vi "BioFeedback12(DoubleEnvelope)-BROKEN.vi"(7 "Frames Per Second":dbl=30.0, 9 "Start Trial":bool, 11 "End Trial":bool, 12 "Data Directory":path, 13 "File Name":string, 14 "Extension":string="_EMG.txt") -> ()   [LabVIEW 2016]
uses:
  <vilib>/Utility/error.llb/DialogType.ctl
  <vilib>/Waveform/WDTOps.llb/WDT Append Waveforms DBL.vi
  <vilib>/Waveform/WDTFileIO.llb/Export Waveforms To Spreadsheet File (1D).vi
  <vilib>/Utility/file.llb/Write Delimited Spreadsheet (string).vi
panel:
  out "frames":dbl
  out "RmsBuffers 2":dbl[][](array[numeric])
  out "rmsBuffersForChannel":dbl[](array[numeric])
  out "romsToAdd":dbl
  out "PrevRMS":dbl
  out "FilteredTrialData":waveform(dbl)[](graph)
  out "FilteredAndRectified":waveform(dbl)[](graph) caption="Filtered and Rectified"
  out "FilteredTrialData":waveform(dbl)[](array[waveform])
  in  "DisplayChannel":dbl
  out "DisplayTrialData":dbl[][](array[numeric])
  out "RMSAverageByChannel":dbl[](array[numeric])
  out "DispBufferSize":dbl
  out "DispBufferIndices":dbl[](array[numeric])
  in  "Big Window Length (s)":dbl=0.5
  out "DisplayBuffers":dbl[][](array[numeric])
  out "ProcessedTrialData":dbl[][](array[numeric])
  out "CurrentRMSByChannel":dbl[](array[numeric])
  out "RmsBuffers":dbl[][](array[numeric])
  out "Trial Data Column Headers":string[](array[string])
  in  "TrialDataRowHeaders":string[](array[string])=["Wfm1", "Wfm2", "Wfm3", "Wfm4", "Wfm5", "Wfm6", "Wfm7", "Wfm8"]
  out "GetMaxStartTime":timestamp
  in  "SecondsToAcquireMax":dbl=10.0
  in  "NumberOfMaximumsToTake":dbl=3.0
  in  "CurrentMaxIndex":dbl
  out "SignalsMaxArray":dbl[](array[numeric])
  out "SignalMaxTrialsArray":dbl[][](array[numeric])
  in  "%StdDevIndex":dbl=5.0
  in  "Mean%Index":dbl=4.0
  in  "StdDevIndex":dbl=3.0
  in  "MeanIndex":dbl=2.0
  in  "MaxIndex":dbl=1.0
  in  "MinIndex":dbl
  out "Stability Data":dbl[][](array[numeric])
  out "RawTrialData":waveform(dbl)[](array[waveform])
  in  "UI Ampl Error Path":path=path "C:/Users/Tinggroup/Desktop/VRMuscleActivationVisualizer/VRBiofeedback_v2/assets/BiofeedbackAmplitudeError.txt"
  out "DisplayActivation":dbl
  out "Acquiring Max":bool
  in  "resetMax":bool
  in  "startGetMax":bool
  in  "Amplitude Error":dbl
  in  "UI Data Path":path=path "C:/Users/Tinggroup/Desktop/VRMuscleActivationVisualizer/VRBiofeedback_v2/assets/LeftEMGData.txt"
  in  "EMG Input Device\nProduct Type":string="USB-6009"
  out "DisplayBarActivation":dbl(slide) caption="Left" max=1.0 scale=0.0..100.0
  out "Processed8":dbl[](graph)
  out "Processsed7":dbl[](graph)
  out "Processed6":dbl[](graph)
  out "Processed5":dbl[](graph)
  out "Processed4":dbl[](graph)
  out "Processed3":dbl[](graph)
  out "Processed2":dbl[](graph)
  out "Processed1":dbl[](graph)
  out "Raw Trial Data Wfm":waveform(dbl)[](graph)
  in  "UI Percent Path":path=path "C:/Users/Tinggroup/Desktop/VRMuscleActivationVisualizer/VRBiofeedback_v2/assets/BiofeedbackTargetPercentage.txt"
  in  "Target Percentage":dbl=10.0
  out "Trial In Progress":bool
  in  "Lower Cut-Off":dbl=20.0
  in  "Upper Cut-Off":dbl=300.0
  out "raw data":dynamicdata(graph)
  out "RmsBufferIndices":dbl[](array[numeric])
  out "RMSBufferSize":dbl
  out "Samples per frame":dbl
  out "Reset Data Acquisition\nAnd UI Updating":bool=TRUE
  in  "Small Window Length (s)":dbl=0.5
  in  "Sample rate (Hz)":dbl=2000.0
  in  "End Program":bool
  # "Saving Trial Data"
  # "Filter and Process Parameters"
  # "Set Target"
  # "Changes are made instantly and cause moving average to reset to zero"
  # "Scale Max"
  # "Channels used in Display"
  # "Analyze Stability of Displayed Data"
  # "Auto Analyze Stability begins calculating stability\nAs soon as dot enters the target zone and stops \nonce the dot leaves the target zone (Not Yet Implemented)"
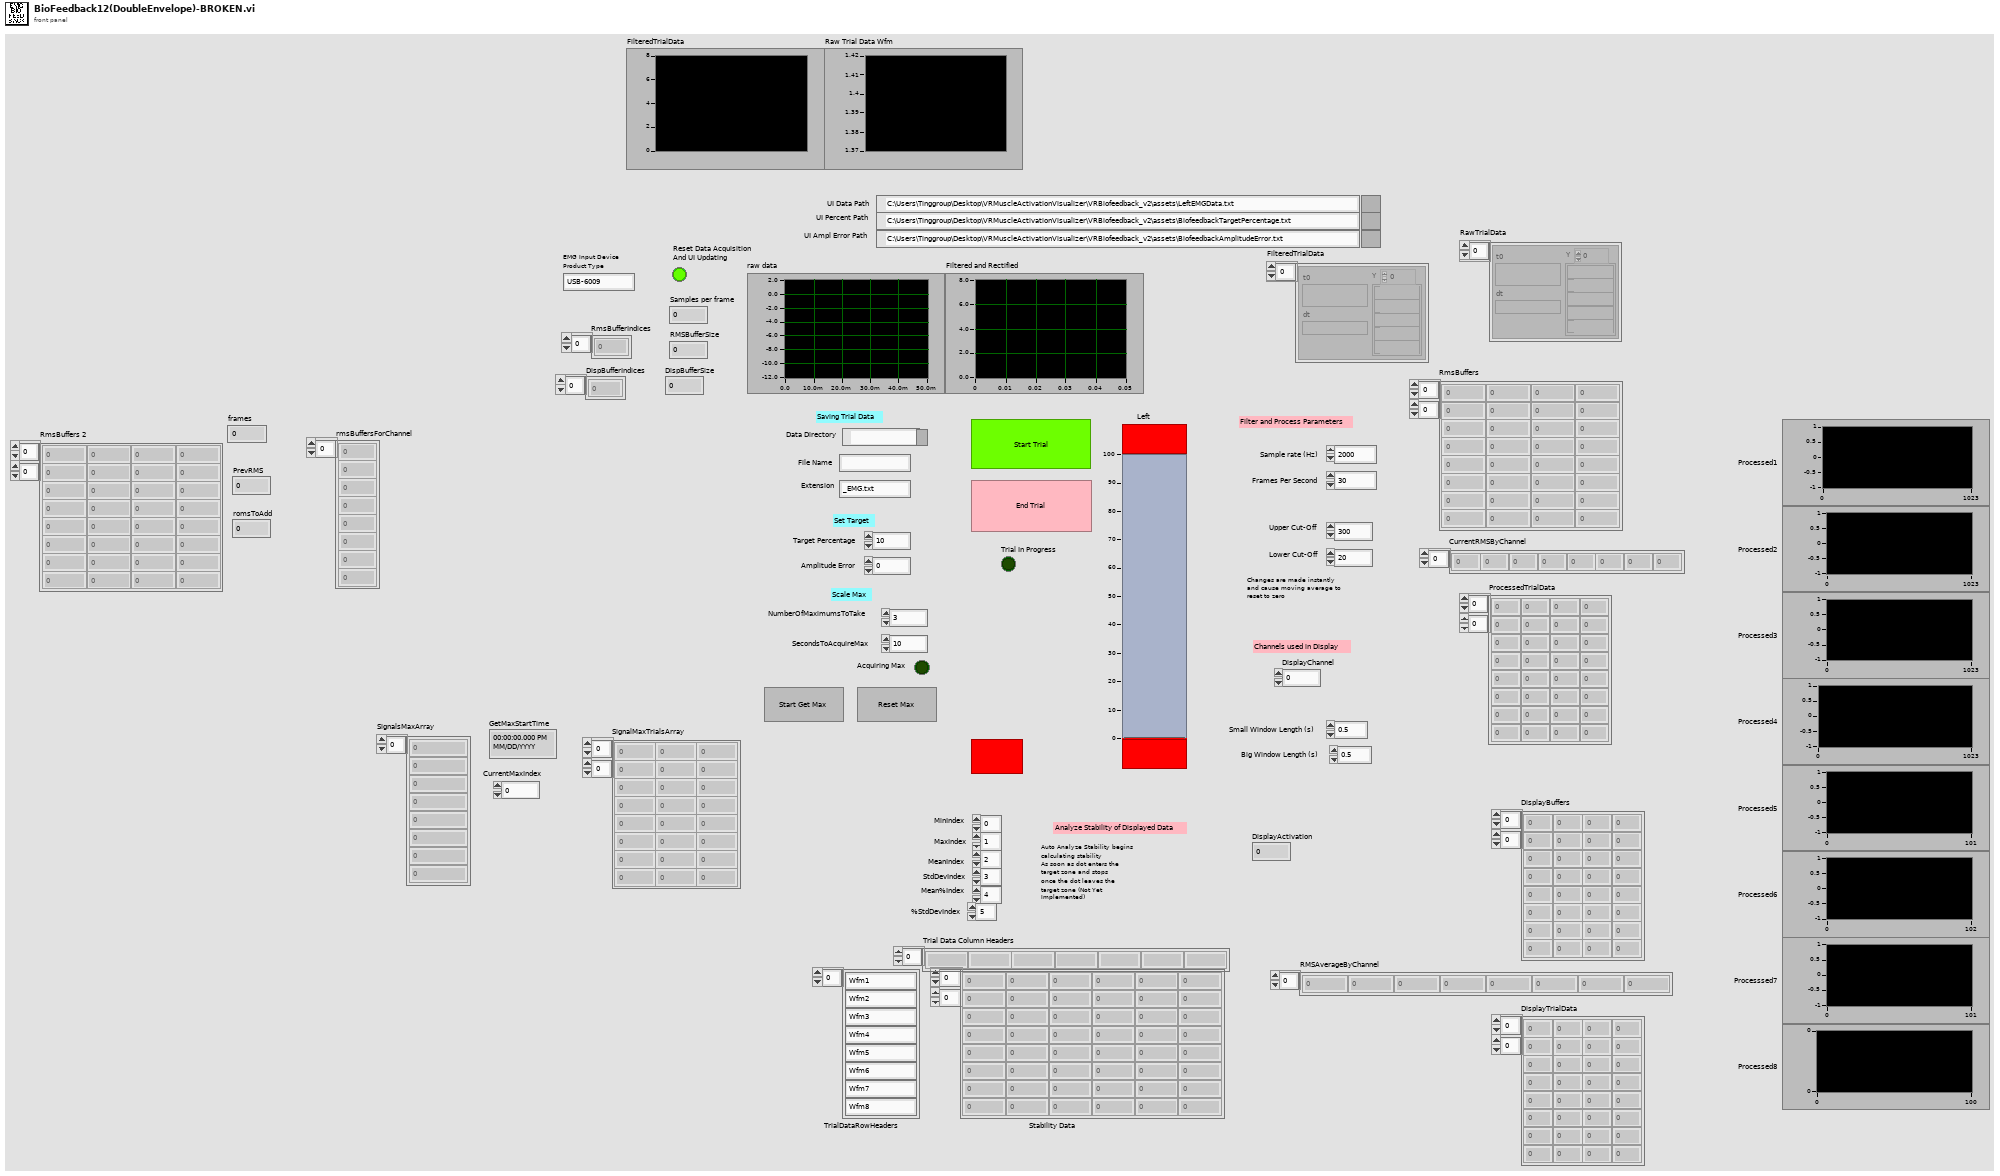
[diagram p1: front panel]
types:
  T1 = typedef "DialogType.ctl" = u16
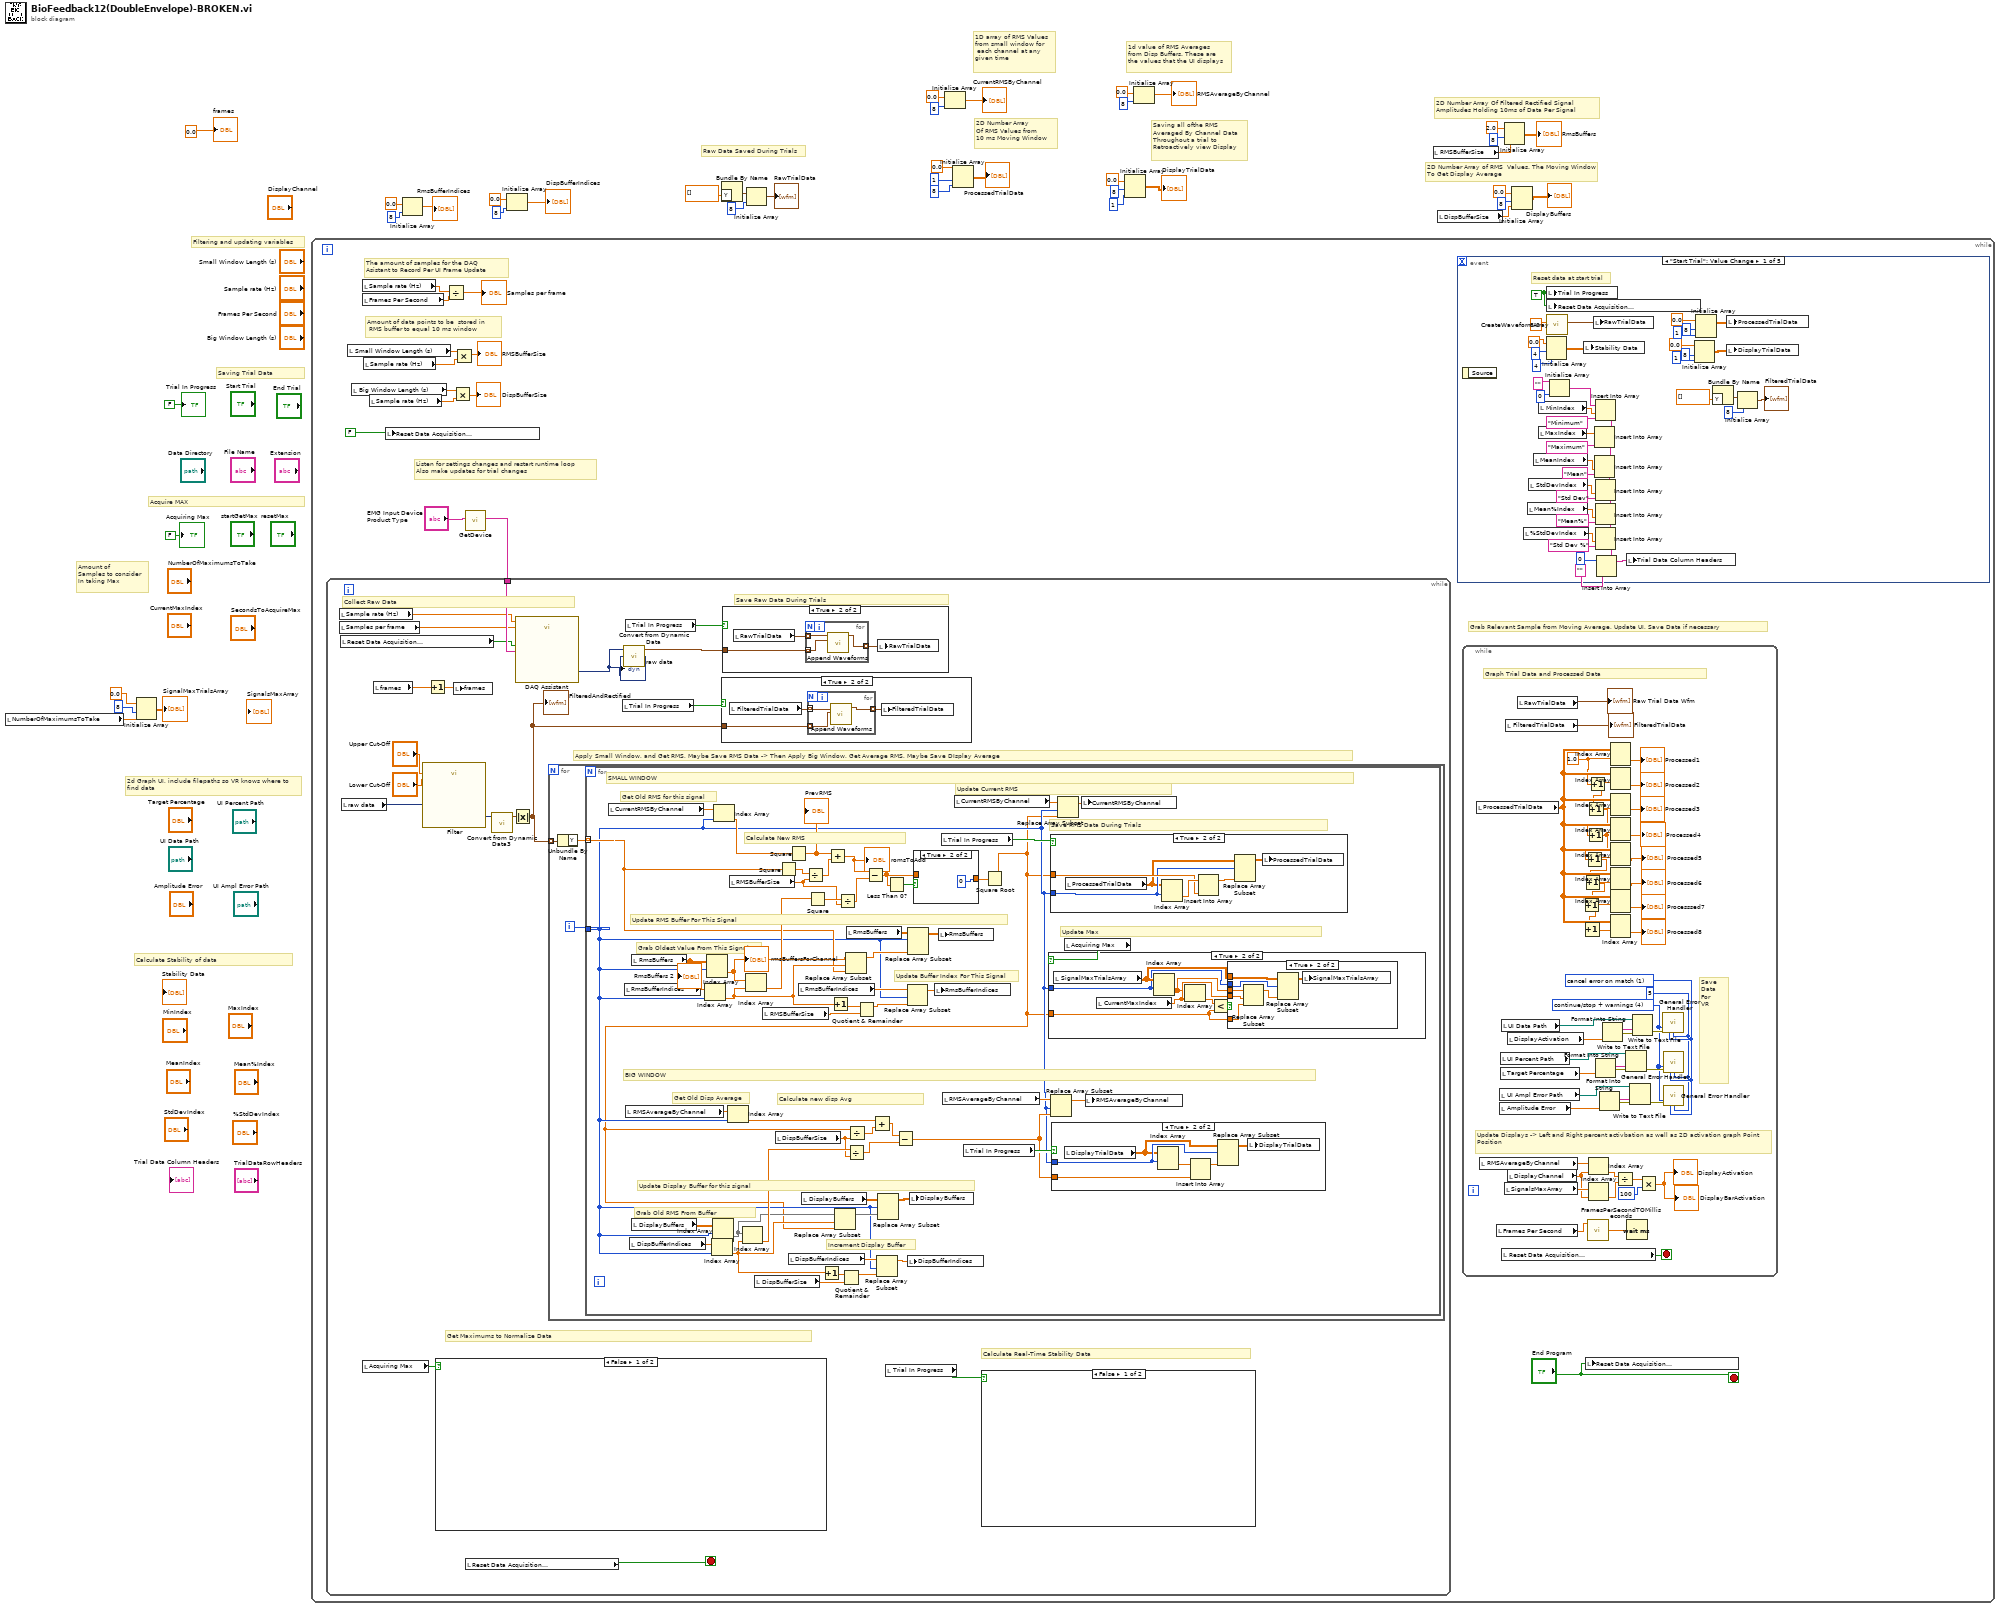
[diagram p0: block diagram]
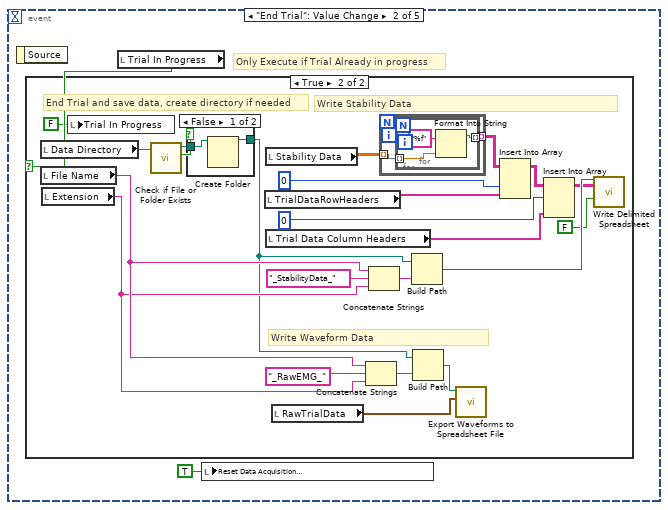
[diagram p2: hidden frame]
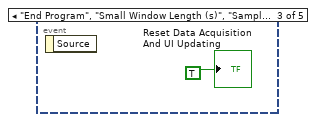
[diagram p5: hidden frame]
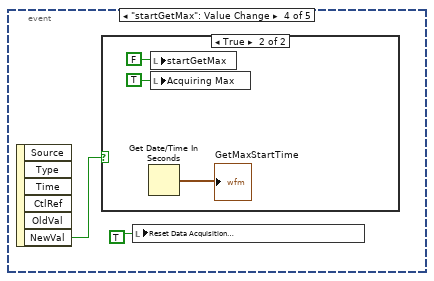
[diagram p6: hidden frame]
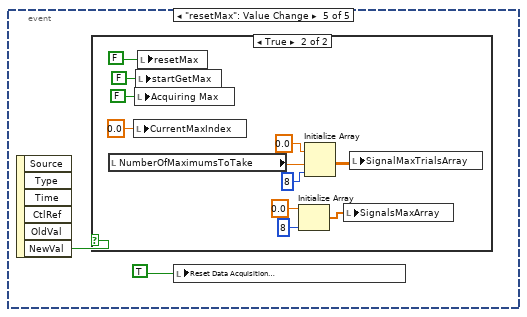
[diagram p8: hidden frame]
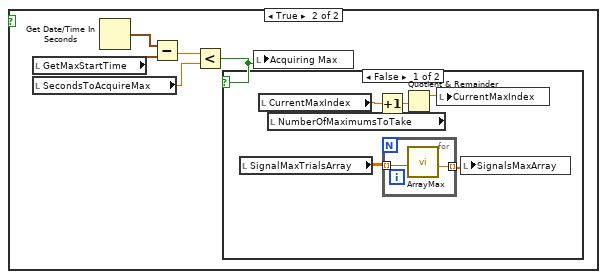
[diagram p17: hidden frame]
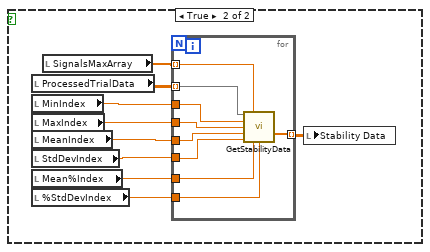
[diagram p19: hidden frame]
diagram:
  # "2D Number Array of RMS  Values. The Moving Window To Get Display Average"
  # "2D Number Array Of Filtered Rectified Signal Amplitudes Holding 10ms of Data Per Signal"
  # "Saving all ofthe RMS\nAveraged By Channel Data\nThroughout a trial to \nRetroactively view Display"
  # "1d value of RMS Averages\nfrom Disp Buffers. These are\nthe values that the UI displays"
  # "1D array of RMS Values\nfrom small window for\n each channel at any\ngiven time"
  # "2D Number Array\nOf RMS Values from\n10 ms Moving Window"
  # "Raw Data Saved During Trials"
  # "Amount of \nSamples to consider\nIn taking Max"
  # "Calculate Stability of data"
  # "Acquire MAX"
  # "Filtering and updating variables"
  # "Saving Trial Data"
  # "2d Graph UI, include filepaths so VR knows where to find data"
  n1 = local read "NumberOfMaximumsToTake"() -> (w13:dbl)
  n2 = Initialize Array(0.0 ("element"), 8 ("dimension size"), w13) -> (→"SignalMaxTrialsArray":dbl[][])
  n3 = while {
    stop <- "End Program" stop-if-true
    # "Amount of data points to be  stored in\n RMS buffer to equal 10 ms window"
    # "Grab Relevant Sample from Moving Average, Update UI, Save Data if necessary"
    # "The amount of samples for the DAQ Asistant to Record Per UI Frame Update"
    # "Listen for settings changes and restart runtime loop\nAlso make updates for trial changes"
    n4 = local read "Small Window Length (s)"() -> (w44:dbl)
    n5 = local read "Big Window Length (s)"() -> (w42:dbl)
    n6 = local read "Sample rate (Hz)"() -> (w52:dbl)
    n7 = local read "Frames Per Second"() -> (w51:dbl)
    n8 = local read "Sample rate (Hz)"() -> (w45:dbl)
    n9 = local read "Sample rate (Hz)"() -> (w41:dbl)
    n10 = local write "Reset Data Acquisition\nAnd UI Updating"(FALSE) -> ()
    n11 = Divide(x=w52, y=w51) -> (x/y=→"Samples per frame":dbl)
    n12 = Multiply(x=w42, y=w41) -> (x*y=→"DispBufferSize":dbl)
    n13 = Multiply(x=w44, y=w45) -> (x*y=→"RMSBufferSize":dbl)
    n14 = call "GetDevice.vi"("EMG Input Device\nProduct Type"="EMG Input Device\nProduct Type") -> ("DAQmx Device Name"=w46:tag)  [unwired: 10 in]
    n15 = while {
      tunnel: w46 -> [w210]
      stop <- w213 stop-if-true
      # "Calculate Real-Time Stability Data"
      # "Get Maximums to Normalize Data"
      # "Save Raw Data During Trials"
      # "Collect Raw Data"
      # "Apply Small Window, and Get RMS, Maybe Save RMS Data -> Then Apply Big Window, Get Average RMS, Maybe Save DIsplay Average"
      n16 = local read "Sample rate (Hz)"() -> (w202:dbl)
      n17 = local read "Samples per frame"() -> (w201:dbl)
      n18 = local read "Reset Data Acquisition\nAnd UI Updating"() -> (w200:bool)
      n19 = local read "raw data"() -> (w214:dynamicdata)
      n20 = local read "Acquiring Max"() -> (w204:bool)
      n21 = local read "frames"() -> (w197:dbl)
      n22 = call "Filter"("Lower Cut-Off"="Lower Cut-Off", "Upper Cut-Off"="Upper Cut-Off", "Signal"=w214) -> ("Filtered Signal"=w212:dynamicdata)  [unwired: 7 in, 1 out]
      n23 = Increment(x=w197) -> (x+1=w196:dbl)
      n24 = case shown="False" w204 {
        frame False {
        }
        frame True {
          n25 = local read "GetMaxStartTime"() -> (w317:timestamp)
          n26 = local read "SecondsToAcquireMax"() -> (w314:dbl)
          n27 = Get Date/Time In Seconds() -> (seconds since 1Jan1904=w316:timestamp)
          n28 = Subtract(x=w316, y=w317) -> (x-y=w315:dbl)
          n29 = Less?(x=w315, y=w314) -> (x < y?=w313:bool)
          n30 = case shown="False" w313 {
            frame False {
              n31 = local read "SignalMaxTrialsArray"() -> (w319:dbl[][])
              n32 = local read "CurrentMaxIndex"() -> (w321:dbl)
              n33 = local read "NumberOfMaximumsToTake"() -> (w323:dbl)
              n34 = Increment(x=w321) -> (x+1=w322:dbl)
              n35 = for {
                tunnel: w319 -> [w325] mode=indexing
                tunnel: [w324] -> w318 mode=indexing
                n36 = call "ArrayMax.vi"("Array"=w325) -> ("max"=w324:dbl)  [unwired: 10 in]
              }
              n37 = Quotient & Remainder(x=w322, y=w323) -> (x-y*floor(x/y)=w320:dbl)  [unwired: 1 out]
              n38 = local write "CurrentMaxIndex"(w320) -> ()
              n39 = local write "SignalsMaxArray"(w318) -> ()
            }
            frame True {
            }
          }
          n40 = local write "Acquiring Max"(w313) -> ()
        }
      }
      n41 = local write "frames"(w196) -> ()
      n42 = local read "Reset Data Acquisition\nAnd UI Updating"() -> (w213:bool)
      n43 = call "Convert from Dynamic Data3"("Dynamic Data Type"=w212) -> ("Array of Waveform"=w211:waveform(dbl)[])  [unwired: 3 in]
      n44 = Absolute Value(x=w211) -> (abs(x)=w198:waveform(dbl)[])
      "FilteredAndRectified" <- w198
      n45 = call "DAQ Assistant"("rate"=w202, "number of samples"=w201, "stop (T)"=w200, "device name"=w210) -> ("data"=w208:dynamicdata)  [unwired: 13 in, 2 out]
      "raw data" <- w208
      n46 = for {
        tunnel: w198 -> [w229] mode=indexing
        i -> [w227]
        n47 = Unbundle By Name(w229) -> ("Y"=w228:dbl[])
        n48 = for {
          tunnel: w228 -> [w239] mode=indexing
          tunnel: w227 -> [w231]
          # "Update Max"
          # "SMALL WINDOW"
          # "BIG WINDOW"
          # "Increment Display Buffer"
          # "Get Old Disp Average"
          # "Calculate new disp Avg"
          # "Grab Old RMS From Buffer"
          # "Update Display Buffer for this signal"
          # "Save RMS Data During Trials"
          # "Update Buffer Index For This Signal"
          # "Update RMS Buffer For This Signal"
          # "Update Current RMS"
          # "Calculate New RMS"
          # "Grab Oldest Value From This Signal"
          # "Get Old RMS for this signal"
          n49 = local read "CurrentRMSByChannel"() -> (w262:dbl[])
          n50 = local read "RmsBufferIndices"() -> (w268:dbl[])
          n51 = local read "RMSAverageByChannel"() -> (w256:dbl[])
          n52 = local read "DispBufferIndices"() -> (w250:dbl[])
          n53 = local read "RmsBuffers"() -> (w263:dbl[][])
          "RmsBuffers 2" <- w263
          n54 = local read "DisplayBuffers"() -> (w259:dbl[][])
          n55 = Index Array(array=w268, index=w231) -> (element=w257:dbl)
          n56 = Index Array(array=w263, index (row)=w231) -> (element=w272:dbl[])  [unwired: 1 in]
          "rmsBuffersForChannel" <- w272
          n57 = Index Array(array=w250, index=w231) -> (element=w242:dbl)
          n58 = Index Array(array=w259, index (row)=w231) -> (element=w236:dbl[])  [unwired: 1 in]
          n59 = Index Array(array=w262, index=w231) -> (element=w277:dbl)
          n60 = Index Array(array=w256, index=w231) -> (element=w247:dbl)
          n61 = local read "RMSBufferSize"() -> (w282:dbl)
          n62 = Index Array(array=w236, index=w242) -> (element=w249:dbl)
          n63 = Index Array(array=w272, index=w257) -> (element=w255:dbl)
          n64 = local read "DispBufferSize"() -> (w261:dbl)
          n65 = local read "RMSBufferSize"() -> (w270:dbl)
          n66 = local read "DispBufferSize"() -> (w246:dbl)
          n67 = Square(x=w239) -> (x^2=w284:dbl)
          n68 = Square(x=w277) -> (x^2=w281:dbl)
          "PrevRMS" <- w281
          n69 = local read "DispBufferIndices"() -> (w241:dbl[])
          n70 = local read "RmsBufferIndices"() -> (w265:dbl[])
          n71 = local read "DisplayBuffers"() -> (w252:dbl[][])
          n72 = Divide(x=w284, y=w282) -> (x/y=w280:dbl)
          n73 = Square(x=w255) -> (x^2=w283:dbl)
          n74 = Increment(x=w242) -> (x+1=w260:dbl)
          n75 = Add(x=w281, y=w280) -> (x+y=w279:dbl)
          "romsToAdd" <- w279
          n76 = Increment(x=w257) -> (x+1=w269:dbl)
          n77 = Divide(x=w283, y=w282) -> (x/y=w278:dbl)
          n78 = Quotient & Remainder(x=w260, y=w261) -> (x-y*floor(x/y)=w240:dbl)  [unwired: 1 out]
          n79 = Replace Array Subset(array=w272, new element=w239, index=w257) -> (w276:dbl[])
          n80 = local read "RmsBuffers"() -> (w273:dbl[][])
          n81 = Divide(x=w249, y=w246) -> (x/y=w253:dbl)
          n82 = Quotient & Remainder(x=w269, y=w270) -> (x-y*floor(x/y)=w266:dbl)  [unwired: 1 out]
          n83 = Subtract(x=w279, y=w278) -> (x-y=w234:dbl)
          n84 = Replace Array Subset(array=w241, new element=w240, index=w231) -> (w238:dbl[])
          n85 = Less Than 0?(x=w234) -> (x < 0?=w235:bool)
          n86 = Replace Array Subset(array=w265, new element=w266, index=w231) -> (w267:dbl[])
          n87 = local write "DispBufferIndices"(w238) -> ()
          n88 = Replace Array Subset(array=w273, new element=w276, index (row)=w231) -> (w271:dbl[][])  [unwired: 1 in]
          n89 = case shown="True" w235 {
            tunnel: w234 -> [w299 _]
            tunnel: [w299 0] -> w233
            frame False {
            }
            frame True {
            }
          }
          n90 = local write "RmsBufferIndices"(w267) -> ()
          n91 = local write "RmsBuffers"(w271) -> ()
          n92 = local read "Trial In Progress"() -> (w264:bool)
          n93 = local read "RMSAverageByChannel"() -> (w245:dbl[])
          n94 = local read "CurrentRMSByChannel"() -> (w275:dbl[])
          n95 = local read "Trial In Progress"() -> (w243:bool)
          n96 = Square Root(x=w233) -> (sqrt(x)=w230:dbl)
          n97 = Replace Array Subset(array=w236, new element=w230, index=w242) -> (w251:dbl[])
          n98 = Divide(x=w230, y=w246) -> (x/y=w248:dbl)
          n99 = Add(x=w247, y=w248) -> (x+y=w254:dbl)
          n100 = Replace Array Subset(array=w252, new element=w251, index (row)=w231) -> (w258:dbl[][])  [unwired: 1 in]
          n101 = Subtract(x=w254, y=w253) -> (x-y=w237:dbl)
          n102 = local write "DisplayBuffers"(w258) -> ()
          n103 = case shown="True" w264 {
            tunnel: w230 -> [_ w309]
            tunnel: w231 -> [_ w308]
            frame False {
            }
            frame True {
              n104 = local read "ProcessedTrialData"() -> (w307:dbl[][])
              n105 = Index Array(array=w307, index (row)=w308) -> (element=w310:dbl[])  [unwired: 1 in]
              n106 = Insert Into Array(array=w310, new element=w309) -> (w311:dbl[])  [unwired: 1 in]
              n107 = Replace Array Subset(array=w307, new element=w311, index (row)=w308) -> (w312:dbl[][])  [unwired: 1 in]
              n108 = local write "ProcessedTrialData"(w312) -> ()
            }
          }
          n109 = Replace Array Subset(array=w245, new element=w237, index=w231) -> (w244:dbl[])
          n110 = case shown="True" w243 {
            tunnel: w231 -> [_ w304]
            tunnel: w237 -> [_ w305]
            frame False {
            }
            frame True {
              n111 = local read "DisplayTrialData"() -> (w303:dbl[][])
              n112 = Index Array(array=w303, index (row)=w304) -> (element=w306:dbl[])  [unwired: 1 in]
              n113 = Insert Into Array(array=w306, new element=w305) -> (w302:dbl[])  [unwired: 1 in]
              n114 = Replace Array Subset(array=w303, new element=w302, index (row)=w304) -> (w301:dbl[][])  [unwired: 1 in]
              n115 = local write "DisplayTrialData"(w301) -> ()
            }
          }
          n116 = Replace Array Subset(array=w275, new element=w230, index=w231) -> (w274:dbl[])
          n117 = local read "Acquiring Max"() -> (w232:bool)
          n118 = case shown="True" w232 {
            tunnel: w231 -> [_ w285]
            tunnel: w230 -> [_ w288]
            frame False {
            }
            frame True {
              n119 = local read "SignalMaxTrialsArray"() -> (w286:dbl[][])
              n120 = local read "CurrentMaxIndex"() -> (w289:dbl)
              n121 = Index Array(array=w286, index (row)=w285) -> (element=w287:dbl[])  [unwired: 1 in]
              n122 = Index Array(array=w287, index=w289) -> (element=w291:dbl)
              n123 = Less?(x=w291, y=w288) -> (x < y?=w290:bool)
              n124 = case shown="True" w290 {
                tunnel: w289 -> [_ w298]
                tunnel: w288 -> [_ w297]
                tunnel: w287 -> [_ w296]
                tunnel: w286 -> [_ w295]
                tunnel: w285 -> [_ w294]
                frame False {
                }
                frame True {
                  n125 = Replace Array Subset(array=w296, new element=w297, index=w298) -> (w293:dbl[])
                  n126 = Replace Array Subset(array=w295, new element=w293, index (row)=w294) -> (w292:dbl[][])  [unwired: 1 in]
                  n127 = local write "SignalMaxTrialsArray"(w292) -> ()
                }
              }
            }
          }
          n128 = local write "CurrentRMSByChannel"(w274) -> ()
          n129 = local write "RMSAverageByChannel"(w244) -> ()
        }
      }
      n130 = local read "Trial In Progress"() -> (w199:bool)
      n131 = call "Convert from Dynamic Data"("Dynamic Data Type"=w208) -> ("Array of Waveform"=w207:waveform(dbl)[])  [unwired: 3 in]
      n132 = local read "Trial In Progress"() -> (w209:bool)
      n133 = case shown="True" w199 {
        tunnel: w198 -> [_ w216]
        frame False {
        }
        frame True {
          n134 = local read "FilteredTrialData"() -> (w217:waveform(dbl)[])
          n135 = for {
            tunnel: w217 -> [w220] mode=indexing
            tunnel: w216 -> [w219] mode=indexing
            tunnel: [w218] -> w215 mode=indexing
            n136 = call-poly <vilib>:"Append Waveforms.vi"("waveform B"=w219, "waveform A"=w220) -> ("waveform out"=w218:waveform(dbl))  [unwired: 8 in, 1 out]
          }
          n137 = local write "FilteredTrialData"(w215) -> ()
        }
      }
      n138 = case shown="True" w209 {
        tunnel: w207 -> [_ w223]
        frame False {
        }
        frame True {
          n139 = local read "RawTrialData"() -> (w222:waveform(dbl)[])
          n140 = for {
            tunnel: w223 -> [w225] mode=indexing
            tunnel: w222 -> [w226] mode=indexing
            tunnel: [w224] -> w221 mode=indexing
            n141 = call-poly <vilib>:"Append Waveforms.vi"("waveform B"=w225, "waveform A"=w226) -> ("waveform out"=w224:waveform(dbl))  [unwired: 8 in, 1 out]
          }
          n142 = local write "RawTrialData"(w221) -> ()
        }
      }
      n143 = local read "Trial In Progress"() -> (w203:bool)
      n144 = case shown="False" w203 {
        frame False {
        }
        frame True {
          n145 = local read "ProcessedTrialData"() -> (w334:dbl[][])
          n146 = local read "MinIndex"() -> (w333:dbl)
          n147 = local read "MaxIndex"() -> (w332:dbl)
          n148 = local read "MeanIndex"() -> (w331:dbl)
          n149 = local read "StdDevIndex"() -> (w330:dbl)
          n150 = local read "Mean%Index"() -> (w329:dbl)
          n151 = local read "%StdDevIndex"() -> (w328:dbl)
          n152 = local read "SignalsMaxArray"() -> (w326:dbl[])
          n153 = for {
            tunnel: w334 -> [w335] mode=indexing
            tunnel: [w336] -> w327 mode=indexing
            tunnel: w333 -> [w343]
            tunnel: w332 -> [w342]
            tunnel: w331 -> [w341]
            tunnel: w330 -> [w340]
            tunnel: w329 -> [w339]
            tunnel: w328 -> [w338]
            tunnel: w326 -> [w337] mode=indexing
            n154 = call "GetStabilityData.vi"("ProvidedData"=w335, "ScaleMax"=w337, "MinIndex"=w343, "MaxIndex"=w342, "MeanIndex"=w341, "StdDevIndex"=w340, "Mean%Index"=w339, "%StdDevIndex"=w338) -> ("ReturnData"=w336:dbl[])  [unwired: 7 in]
          }
          n155 = local write "Stability Data"(w327) -> ()
        }
      }
    }
    n156 = event shown="[0] \"Start Trial\": Value Change" {
      selector: _ -> [_ _ _ _ _]
      dyn-events: _ -> [_ _ _ _ _]
      timeout: _ -> [_ _ _ _ _]
      event "Start Trial": Value Change {
        w95 = TRUE ("Trial In Progress")
        # "Reset data at start trial"
        n157 = event-data() -> ()  [unwired: 1 in, 1 out]
        n158 = local read "%StdDevIndex"() -> (w71:dbl)
        n159 = local read "Mean%Index"() -> (w72:dbl)
        n160 = local read "StdDevIndex"() -> (w76:dbl)
        n161 = local read "MeanIndex"() -> (w80:dbl)
        n162 = local read "MaxIndex"() -> (w83:dbl)
        n163 = local read "MinIndex"() -> (w85:dbl)
        n164 = Initialize Array(0.0 ("element"), 4 ("dimension size"), 4 ("dimension size")) -> (w89:dbl[][])
        n165 = local write "Trial In Progress"(w95) -> ()
        n166 = local write "Reset Data Acquisition\nAnd UI Updating"(w95) -> ()
        n167 = call "CreateWaveformArray.vi"("bufferSize"=8.0) -> ("initialized array"=w94:waveform(dbl)[])  [unwired: 5 in, 1 out]
        n168 = Initialize Array("", 0 ("dimension size")) -> (w84:string[])
        n169 = local write "Stability Data"(w89) -> ()
        n170 = local write "RawTrialData"(w94) -> ()
        n171 = Insert Into Array(array=w84, index=w85, new element="Minimum" ("new element/subarray")) -> (w81:string[])
        n172 = Insert Into Array(array=w81, index=w83, new element="Maximum" ("new element/subarray")) -> (w78:string[])
        n173 = Insert Into Array(array=w78, index=w80, new element="Mean" ("new element/subarray")) -> (w75:string[])
        n174 = Insert Into Array(array=w75, index=w76, new element="Std Dev" ("new element/subarray")) -> (w73:string[])
        n175 = Insert Into Array(array=w73, index=w72, new element="Mean%" ("new element/subarray")) -> (w69:string[])
        n176 = Insert Into Array(array=w69, index=w71, new element="Std Dev %" ("new element/subarray")) -> (w66:string[])
        n177 = Insert Into Array(array=w66, index=0, new element="" ("new element/subarray")) -> (w67:string[])
        n178 = local write "Trial Data Column Headers"(w67) -> ()
        n179 = Initialize Array(0.0 ("element"), 8 ("dimension size"), 1 ("dimension size")) -> (w57:dbl[][])
        n180 = Initialize Array(0.0 ("element"), 8 ("dimension size"), 1 ("dimension size")) -> (w64:dbl[][])
        n181 = Bundle By Name("Y"=dbl[] []) -> (w55:waveform(dbl))  [unwired: 1 in]
        n182 = local write "ProcessedTrialData"(w64) -> ()
        n183 = local write "DisplayTrialData"(w57) -> ()
        n184 = Initialize Array(w55, 8 ("dimension size")) -> (→"FilteredTrialData":waveform(dbl)[])
      }
      event "End Trial": Value Change {
        # "Only Execute if Trial Already in progress"
        n185 = event-data() -> ()  [unwired: 1 in, 1 out]
        n186 = local read "Trial In Progress"() -> (w97:bool)
        n187 = case shown="True" w97 {
          frame False {
          }
          frame True {
            # "Write Waveform Data"
            # "Write Stability Data"
            # "End Trial and save data, create directory if needed"
            n188 = local read "Data Directory"() -> (w117:path)
            n189 = local read "File Name"() -> (w103:string)
            n190 = local read "Extension"() -> (w102:string)
            n191 = local write "Trial In Progress"(FALSE ("Trial In Progress")) -> ()
            n192 = call <vilib>:"Check if File or Folder Exists.vi"("path"=w117) -> ("file or folder exists?"=w119:bool, "dup path"=w118:path)  [unwired: 8 in, 1 out]
            n193 = case shown="False" w119 {
              tunnel: [w126 w128] -> w101
              tunnel: w118 -> [w127 w128]
              frame False {
                n194 = Create Folder(path (use dialog)=w127) -> (created path=w126:path)  [unwired: 2 in, 2 out]
              }
              frame True {
              }
            }
            n195 = local read "TrialDataRowHeaders"() -> (w112:string[])
            n196 = local read "Stability Data"() -> (w109:dbl[][])
            n197 = local read "Trial Data Column Headers"() -> (w113:string[])
            n198 = local read "RawTrialData"() -> (w99:waveform(dbl)[])
            n199 = Concatenate Strings(w103, "_RawEMG_" ("string"), w102) -> (w100:string)
            n200 = Concatenate Strings(w103, "_StabilityData_" ("string"), w102) -> (w105:string)
            n201 = for {
              tunnel: w109 -> [w122] mode=indexing
              tunnel: [w121] -> w107 mode=indexing
              n202 = for {
                tunnel: w122 -> [w124] mode=indexing
                tunnel: [w123] -> w121 mode=indexing
                n203 = Format Into String(format string="%f", w124) -> (resulting string=w123:string)  [unwired: 2 in, 1 out]
              }
            }
            n204 = Build Path(base path=w101, name or relative path=w105) -> (appended path=w115:path)
            n205 = Build Path(base path=w101, name or relative path=w100) -> (appended path=w98:path)
            n206 = call-poly <vilib>:"Export Waveforms to Spreadsheet File.vi"("waveforms"=w99, "file path (dialog if empty)"=w98) -> ()  [unwired: 8 in, 2 out]
            n207 = Insert Into Array(array=w107, index (col)=0 ("index (row)"), new element=w112) -> (w116:string[][])  [unwired: 1 in]
            n208 = Insert Into Array(array=w116, index (row)=0 ("index (col)"), new element=w113) -> (w108:string[][])  [unwired: 1 in]
            n209 = call-poly <vilib>:"Write Delimited Spreadsheet.vi"("file path (dialog if empty)"=w115, "2D data"=w108, "append to file? (new file:F)"=FALSE) -> ()  [unwired: 11 in, 2 out]
          }
        }
        n210 = local write "Reset Data Acquisition\nAnd UI Updating"(TRUE ("Reset Data Acquisition\nAnd UI Updating")) -> ()
      }
      event "End Program", "Small Window Length (s)", "Sample rate (Hz)", "Frames Per Second": Value Change {
        n211 = event-data() -> ()  [unwired: 1 in, 1 out]
        "Reset Data Acquisition\nAnd UI Updating" <- TRUE
      }
      event "startGetMax": Value Change {
        n212 = event-data() -> ("NewVal"=w131:bool)  [unwired: 1 in, 5 out]
        n213 = case shown="True" w131 {
          frame False {
          }
          frame True {
            n214 = Get Date/Time In Seconds() -> (seconds since 1Jan1904=→"GetMaxStartTime":timestamp)
            n215 = local write "startGetMax"(FALSE) -> ()
            n216 = local write "Acquiring Max"(TRUE ("Acquiring Max")) -> ()
          }
        }
        n217 = local write "Reset Data Acquisition\nAnd UI Updating"(TRUE ("Reset Data Acquisition\nAnd UI Updating")) -> ()
      }
      event "resetMax": Value Change {
        n218 = event-data() -> ("NewVal"=w136:bool)  [unwired: 1 in, 5 out]
        n219 = case shown="True" w136 {
          frame False {
          }
          frame True {
            n220 = local read "NumberOfMaximumsToTake"() -> (w142:dbl)
            n221 = local write "CurrentMaxIndex"(0.0 ("CurrentMaxIndex")) -> ()
            n222 = local write "Acquiring Max"(FALSE ("Acquiring Max")) -> ()
            n223 = local write "startGetMax"(FALSE ("startGetMax")) -> ()
            n224 = local write "resetMax"(FALSE ("endGetMax")) -> ()
            n225 = Initialize Array(0.0 ("element"), 8 ("dimension size")) -> (w138:dbl[])
            n226 = Initialize Array(0.0 ("element"), w142, 8 ("dimension size")) -> (w143:dbl[][])
            n227 = local write "SignalsMaxArray"(w138) -> ()
            n228 = local write "SignalMaxTrialsArray"(w143) -> ()
          }
        }
        n229 = local write "Reset Data Acquisition\nAnd UI Updating"(TRUE ("Reset Data Acquisition\nAnd UI Updating")) -> ()
      }
    }
    n230 = while {
      stop <- w195 stop-if-true
      w154 = 1.0 ("x")
      w174 = T1 4 items=["no dialog", "OK message", "continue or stop message", "OK message + warnings", "continue/stop + warnings"] ("type of dialog (OK msg:1)")
      w173 = 1 items=["no exception", "cancel error on match", "set error on match"] ("[exception action] (none:0)")
      w172 = 5 ("[exception code]")
      # "Graph Trial Data and Processed Data"
      # "Update Displays -> Left and Right percent activbation as well as 2D activation graph Point Position"
      # "Save\nData\nFor\nVR"
      n231 = local read "ProcessedTrialData"() -> (w163:dbl[][])
      n232 = local read "RMSAverageByChannel"() -> (w153:dbl[])
      n233 = local read "Frames Per Second"() -> (w194:dbl)
      n234 = local read "UI Ampl Error Path"() -> (w175:path)
      n235 = local read "Amplitude Error"() -> (w176:dbl)
      n236 = local read "UI Percent Path"() -> (w184:path)
      n237 = local read "Target Percentage"() -> (w183:dbl)
      n238 = local read "UI Data Path"() -> (w191:path)
      n239 = local read "Reset Data Acquisition\nAnd UI Updating"() -> (w195:bool)
      n240 = local read "SignalsMaxArray"() -> (w152:dbl[])
      n241 = local read "FilteredTrialData"() -> (→"FilteredTrialData":waveform(dbl)[])
      n242 = local read "DisplayActivation"() -> (w189:dbl)
      n243 = local read "DisplayChannel"() -> (w151:dbl)
      n244 = local read "RawTrialData"() -> (→"Raw Trial Data Wfm":waveform(dbl)[])
      n245 = Increment(x=w154) -> (x+1=w155:dbl)
      n246 = Increment(x=w155) -> (x+1=w156:dbl)
      n247 = Increment(x=w156) -> (x+1=w157:dbl)
      n248 = Increment(x=w157) -> (x+1=w158:dbl)
      n249 = Increment(x=w158) -> (x+1=w159:dbl)
      n250 = Increment(x=w159) -> (x+1=w160:dbl)
      n251 = Increment(x=w160) -> (x+1=w161:dbl)
      n252 = call "FramesPerSecondTOMilliseconds.vi"("Thermometer\nFps"=w194) -> ("x*y"=w171:dbl)  [unwired: 10 in]
      n253 = Index Array(array=w153, index=w151) -> (element=w150:dbl)
      n254 = Index Array(array=w152, index=w151) -> (element=w149:dbl)
      n255 = Format Into String(w183) -> (resulting string=w185:string, error out=w186:errorcluster)  [unwired: 3 in]
      n256 = Format Into String(w176) -> (resulting string=w177:string, error out=w178:errorcluster)  [unwired: 3 in]
      n257 = Format Into String(w189) -> (resulting string=w190:string, error out=w192:errorcluster)  [unwired: 3 in]
      n258 = Index Array(array=w163, index (row)=w154) -> (element=→"Processed1":dbl[])  [unwired: 1 in]
      n259 = Index Array(array=w163, index (row)=w155) -> (element=→"Processed2":dbl[])  [unwired: 1 in]
      n260 = Index Array(array=w163, index (row)=w156) -> (element=→"Processed3":dbl[])  [unwired: 1 in]
      n261 = Index Array(array=w163, index (row)=w157) -> (element=→"Processed4":dbl[])  [unwired: 1 in]
      n262 = Index Array(array=w163, index (row)=w158) -> (element=→"Processed5":dbl[])  [unwired: 1 in]
      n263 = Index Array(array=w163, index (row)=w159) -> (element=→"Processed6":dbl[])  [unwired: 1 in]
      n264 = Index Array(array=w163, index (row)=w160) -> (element=→"Processsed7":dbl[])  [unwired: 1 in]
      n265 = Index Array(array=w163, index (row)=w161) -> (element=→"Processed8":dbl[])  [unwired: 1 in]
      n266 = Divide(x=w150, y=w149) -> (x/y=w181:dbl)
      n267 = Write to Text File(file (use dialog)=w184, text=w185, error in=w186) -> (error out=w187:errorcluster)  [unwired: 1 in, 2 out]
      n268 = Wait (ms)(milliseconds to wait=w171) -> ()  [unwired: 1 out]
      n269 = Write to Text File(file (use dialog)=w175, text=w177, error in=w178) -> (error out=w179:errorcluster)  [unwired: 1 in, 2 out]
      n270 = Write to Text File(file (use dialog)=w191, text=w190, error in=w192) -> (error out=w193:errorcluster)  [unwired: 1 in, 2 out]
      n271 = Multiply(x=w181, y=100) -> (x*y=→"DisplayBarActivation" →"DisplayActivation":dbl)
      n272 = call <vilib>:"General Error Handler.vi"("type of dialog (OK msg:1)"=w174, "error in (no error)"=w193, "[exception action] (none:0)"=w173, "[exception code]"=w172) -> ()  [unwired: 7 in, 5 out]
      n273 = call <vilib>:"General Error Handler.vi"("type of dialog (OK msg:1)"=w174, "error in (no error)"=w187, "[exception action] (none:0)"=w173, "[exception code]"=w172) -> ()  [unwired: 7 in, 5 out]
      n274 = call <vilib>:"General Error Handler.vi"("type of dialog (OK msg:1)"=w174, "error in (no error)"=w179, "[exception action] (none:0)"=w173, "[exception code]"=w172) -> ()  [unwired: 7 in, 5 out]
    }
    n275 = local write "Reset Data Acquisition\nAnd UI Updating"("End Program") -> ()
  }
  n276 = Initialize Array(0.0 ("element"), 8 ("dimension size")) -> (→"RmsBufferIndices":dbl[])
  n277 = Initialize Array(0.0 ("element"), 8 ("dimension size")) -> (→"DispBufferIndices":dbl[])
  n278 = Bundle By Name("Y"=dbl[] []) -> (w18:waveform(dbl))  [unwired: 1 in]
  n279 = Initialize Array(w18, 8 ("dimension size")) -> (→"RawTrialData":waveform(dbl)[])
  n280 = Initialize Array(0.0 ("element"), 8 ("dimension size")) -> (→"CurrentRMSByChannel":dbl[])
  n281 = Initialize Array(0.0 ("element"), 1 ("dimension size"), 8 ("dimension size")) -> (→"ProcessedTrialData":dbl[][])
  n282 = Initialize Array(0.0 ("element"), 8 ("dimension size"), 1 ("dimension size")) -> (→"DisplayTrialData":dbl[][])
  n283 = Initialize Array(0.0 ("element"), 8 ("dimension size")) -> (→"RMSAverageByChannel":dbl[])
  n284 = local read "RMSBufferSize"() -> (w12:dbl)
  n285 = local read "DispBufferSize"() -> (w11:dbl)
  n286 = Initialize Array(2.0 ("element"), 8 ("dimension size"), w12) -> (→"RmsBuffers":dbl[][])
  n287 = Initialize Array(0.0 ("element"), 8 ("dimension size"), w11) -> (→"DisplayBuffers":dbl[][])
  "Trial In Progress" <- FALSE ("Trial In Progress")
  "Acquiring Max" <- FALSE ("Acquiring Max")
  "frames" <- 0.0 ("frames")
